vi "Get Clients.vi"(8 "error in":errorcluster, 11 "System in":refnum<class "System.lvclass">) -> (0 "error out":errorcluster, 3 "System out":refnum<class "System.lvclass">)   [LabVIEW 2014, in "System.lvclass"]
uses:
  System.lvclass
  Controls/Client Ref.ctl
  <vilib>/xml/Close Reference(Node).vi
  <vilib>/xml/Close Reference(NNMap).vi
  <vilib>/xml/NI_XML.lvlib
  <resource>/objmgr/DOMUserDefRef.rc
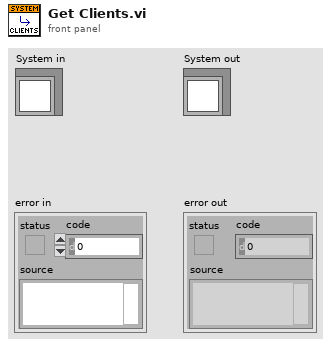
[diagram p1: front panel]
types:
  T1 = typedef "Client Ref.ctl" = cluster{"Name":string, "Path":path}
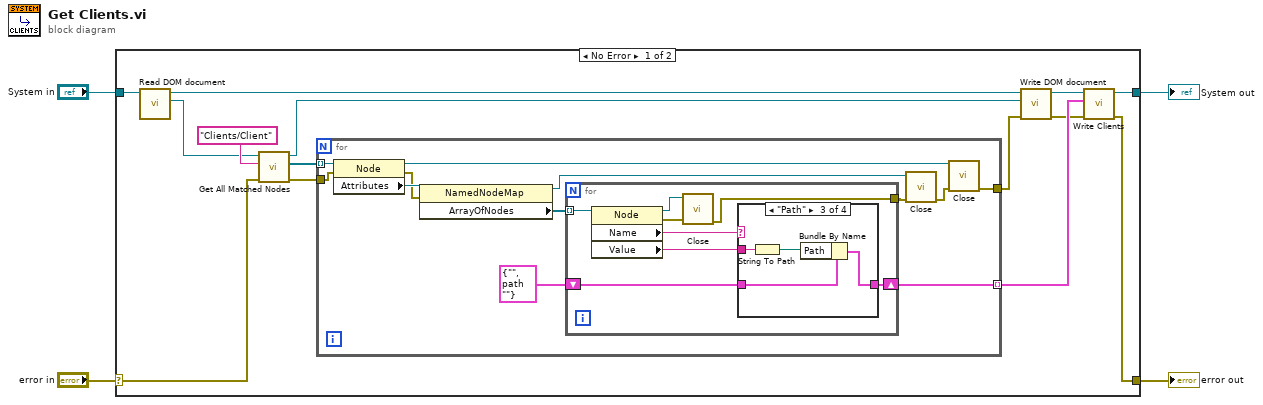
[diagram p0: block diagram]
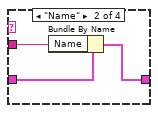
[diagram p3: hidden frame]
diagram:
  n1 = case shown="No Error" "error in" {
    selector: "error in" -> [w17 w49]
    tunnel: [w5 w49] -> w3
    tunnel: [w16 w48] -> w1
    tunnel: "System in" -> [w15 w48]
    frame No Error {
      n2 = call-dynamic "Read DOM document.vi"("System in"=w15) -> ("DOM document"=w8:refnum<k20>, "System out"=w12:refnum<class "System.lvclass">)  [unwired: 8 in, 1 out]
      n3 = call <vilib>:"Get All Matched Nodes.vi"("error in (no error)"=w17, "XPath expression"="Clients/Client", "node in"=w8) -> ("error out"=w13:errorcluster, "node result array"=w14:refnum<k20>[], "node out"=w7:refnum<k20>)  [unwired: 6 in]
      n4 = for {
        tunnel: w14 -> [w30] mode=indexing
        tunnel: w13 -> [w28]
        tunnel: [w24] -> w11 mode=indexing
        tunnel: [w19] -> w9
        n5 = property class="Node"(reference=w30, error in=w28) -> (reference out=w20:refnum<k20>, error out=w27:errorcluster, "Attributes"=w29:refnum<k20>)
        n6 = property class="NamedNodeMap"(reference=w29, error in=w27) -> (reference out=w22:refnum<k20>, "ArrayOfNodes"=w26:refnum<k20>[])  [unwired: 1 out]
        n7 = for {
          tunnel: w26 -> [w38] mode=indexing
          shift-right: [w32] -> w24
          shift-left: T1 {"Name"="", "Path"=path ""} ("Client") -> [w33]
          tunnel: [w31] -> w23
          n8 = property class="Node"(reference=w38) -> (reference out=w36:refnum<k20>, error out=w37:errorcluster, "Name"=w35:string, "Value"=w34:string)  [unwired: 1 in]
          n9 = call-poly <vilib>:"Close.vi"("error in (no error)"=w37, "node"=w36) -> ("error out"=w31:errorcluster)  [unwired: 7 in]
          n10 = case shown="\"Path\"" w35 {
            tunnel: w34 -> [_ w41 w46 _]
            tunnel: w33 -> [w39 w42 w45 w47]
            tunnel: [w39 w40 w43 w47] -> w32
            frame Default {
              # "Error in config"
            }
            frame "Name" {
              n11 = Bundle By Name(cluster=w42, "Name"=w41) -> (w40:T1)
            }
            frame "Path" {
              n12 = String To Path(string=w46) -> (path=w44:path)
              n13 = Bundle By Name(cluster=w45, "Path"=w44) -> (w43:T1)
            }
            frame "InitializationData" {
              # "Can add later"
            }
          }
        }
        n14 = call-poly <vilib>:"Close.vi"("error in (no error)"=w23, "named node map"=w22) -> ("error out"=w21:errorcluster)  [unwired: 7 in]
        n15 = call-poly <vilib>:"Close.vi"("error in (no error)"=w21, "node"=w20) -> ("error out"=w19:errorcluster)  [unwired: 7 in]
      }
      n16 = call-dynamic "Write DOM document.vi"("error in"=w9, "DOM document"=w7, "System in"=w12) -> ("error out"=w6:errorcluster, "System out"=w10:refnum<class "System.lvclass">)  [unwired: 7 in]
      n17 = call-dynamic "Write Clients.vi"("error in"=w6, "Clients"=w11, "System in"=w10) -> ("error out"=w5:errorcluster, "System out"=w16:refnum<class "System.lvclass">)  [unwired: 7 in]
    }
    frame Error {
    }
  }
  "error out" <- w3
  "System out" <- w1
